vi "Handle Received Heartbeat Message.vi"(8 "error in":errorcluster, 10 "CANopen Message":refnum<class "CANopen Response Message.lvclass">, 11 "CANopen Master in":refnum<class "CANopen Master.lvclass">) -> (0 "error out":errorcluster, 3 "CANopen Master out":refnum<class "CANopen Master.lvclass">)   [LabVIEW 2024, in "CANopen Master.lvclass"]
doc: "Handles a received NMT Message. Resets an awaited heartbeat. Extracts Sender's state and fires a Node Discovered event in case a new node is on the bus."
uses:
  CANopen Master.lvclass
  CANopen Response/CANopen Response Message.lvclass
  CANopen Master.lvclass/CANopen Master.ctl
  Example/Network Management/Network Mangement.lvclass
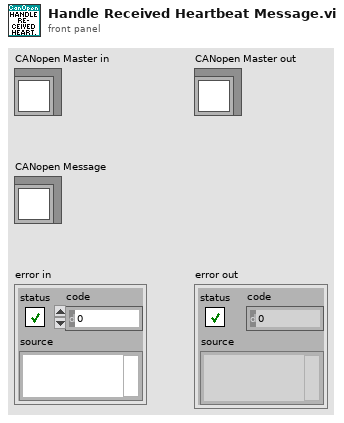
[diagram p1: front panel]
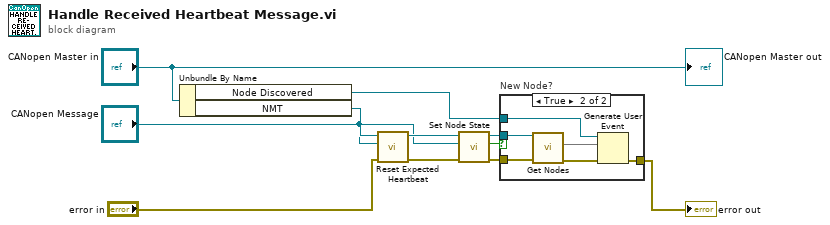
[diagram p0: block diagram]
diagram:
  n1 = Unbundle By Name("CANopen Master in") -> ("Node Discovered"=w4:refnum<user-event>, "NMT"=w3:refnum<class "Network Mangement.lvclass">)
  n2 = call "Reset Expected Heartbeat.vi"("Error In"="error in", "CANopen Message"="CANopen Message", "reference in"=w3) -> ("Error Out"=w8:errorcluster, "reference out"=w2:refnum<class "Network Mangement.lvclass">)  [unwired: 7 in]
  n3 = call "Set Node State.vi"("Error In"=w8, "CANopen Message"="CANopen Message", "reference in"=w2) -> ("Error Out"=w11:errorcluster, "New Node/State?"=w6:bool, "reference out"=w5:refnum<class "Network Mangement.lvclass">)  [unwired: 6 in]
  n4 = case "New Node?" shown="True" w6 {
    tunnel: w11 -> [w12 w18]
    tunnel: w5 -> [_ w15]
    tunnel: w4 -> [_ w13]
    tunnel: [w12 w16] -> w10
    frame False {
    }
    frame True {
      n5 = call "Get Nodes.vi"("Error In"=w18, "reference in"=w15) -> ("Error Out"=w17:errorcluster, "Nodes"=w14:map{u8, u8})  [unwired: 7 in, 1 out]
      n6 = Generate User Event(user event=w13, event data cluster=w14, error in=w17) -> (error out=w16:errorcluster)  [unwired: 1 in, 1 out]
    }
  }
  "error out" <- w10
  "CANopen Master out" <- "CANopen Master in"
